vi "Test Basic Function 6.vi"() -> ()   [LabVIEW 2014]
uses:
  Arduino Math.lvlib
panel:
  out "Error Out":errorcluster
  out "pow(x,y)":sgl
  out "log10(x)":sgl
  out "log(x)":sgl
  in  "Error In":errorcluster
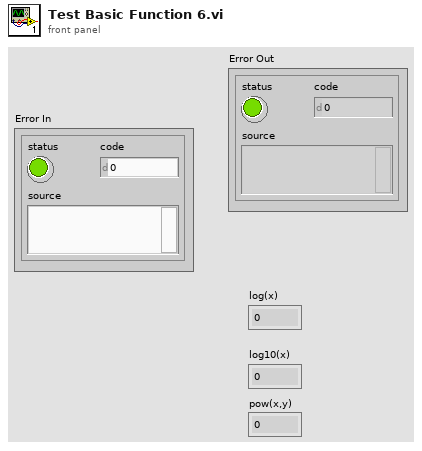
[diagram p1: front panel]
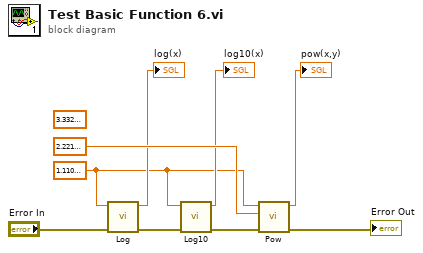
[diagram p0: block diagram]
diagram:
  (unwired) sgl 3.333 ("x")
  w2 = sgl 1.111 ("x")
  n1 = call "Log.vi"("Error In"="Error In", "x"=w2) -> ("Error Out"=w7:errorcluster, "log(x)"=→"log(x)":sgl)  [unwired: 8 in]
  n2 = call "Log10.vi"("Error In"=w7, "x"=w2) -> ("Error Out"=w6:errorcluster, "log10(x)"=→"log10(x)":sgl)  [unwired: 8 in]
  n3 = call "Pow.vi"("Error In"=w6, "y"=sgl 2.222 ("x"), "x"=w2) -> ("Error Out"=→"Error Out":errorcluster, "pow(x,y)"=→"pow(x,y)":sgl)  [unwired: 7 in]
